vi "2B Dialog with Font Size control.vi"(8 "error in (no error)":errorcluster, 9 "F Button Name (\"Cancel\")":string="Cancel", 10 "T Button Name (\"OK\")":string="Retry", 11 "message":string="System On Signal Not Received.\nPlease TURN ON the System On Switch On the Front Door.") -> (0 "error out":errorcluster, 3 "OK":bool)   [LabVIEW 2018]
panel:
  out "message":string
  in  "OK":bool
  in  "Cancel":bool
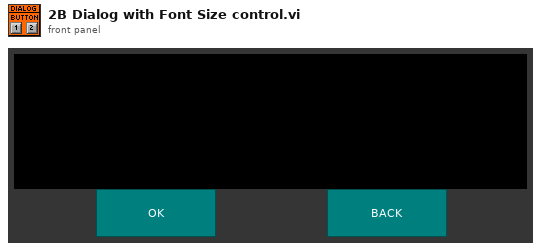
[diagram p1: front panel]
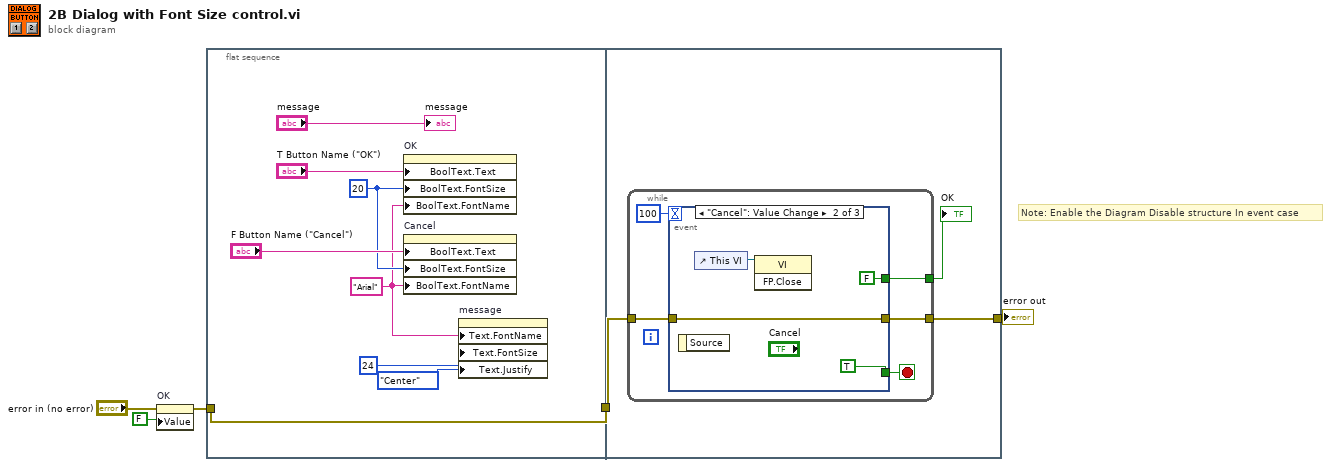
[diagram p0: block diagram]
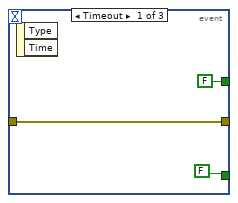
[diagram p2: hidden frame]
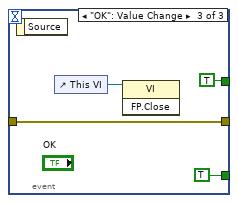
[diagram p3: hidden frame]
diagram:
  # "Note: Enable the Diagram Disable structure In event case"
  n1 = property on="OK" class="Bool (strict)"(error in="error in (no error)", "Value"=FALSE ("OK")) -> (error out=w2:errorcluster)  [unwired: 1 in, 1 out]
  n2 = flat-sequence {
    tunnel: [w10] -> w5
    tunnel: w2 -> [w10]
    tunnel: w5 -> [w15]
    tunnel: [w14] -> w4
    frame #0 {
      w7 = "Arial" ("Font Name")
      w11 = u32 20 ("Boolean Text.Font:Size")
      n3 = property on="OK" class="Bool"("BoolText.Text"="T Button Name (\"OK\")", "BoolText.FontSize"=w11, "BoolText.FontName"=w7) -> ()  [unwired: 2 in, 2 out]
      n4 = property on="Cancel" class="Bool"("BoolText.Text"="F Button Name (\"Cancel\")", "BoolText.FontSize"=w11, "BoolText.FontName"=w7) -> ()  [unwired: 2 in, 2 out]
      n5 = property on="message" class="Str"("Text.FontName"=w7, "Text.FontSize"=u32 24 ("Text.Font:Size"), "Text.Justify"=enum16{"Left", "Center", "Right"}."Center" ("Text.Justification")) -> ()  [unwired: 2 in, 2 out]
      "message" <- "message"
    }
    frame #1 {
      n6 = while {
        tunnel: [w19] -> w16
        tunnel: w15 -> [w17]
        tunnel: [w18] -> w14
        stop <- w20 stop-if-true
        n7 = event shown="[1] \"Cancel\": Value Change" {
          selector: _ -> [_ _ _]
          dyn-events: _ -> [_ _ _]
          timeout: 100 -> [_ _ _]
          tunnel: [FALSE TRUE TRUE] -> w20
          tunnel: [FALSE FALSE TRUE] -> w19
          tunnel: [w22 w26 w30] -> w18
          tunnel: w17 -> [w22 w26 w30]
          event Timeout {
            n8 = event-data() -> ()  [unwired: 3 out]
          }
          event "Cancel": Value Change {
            n9 = event-data() -> ()  [unwired: 2 out]
            n10 = control-ref of="This VI"() -> (w25:refnum<vi>)
            n11 = invoke class="VI" method="FP.Close"(reference=w25) -> ()  [unwired: 2 in, 3 out]
          }
          event "OK": Value Change {
            n12 = event-data() -> ()  [unwired: 2 out]
            n13 = control-ref of="This VI"() -> (w29:refnum<vi>)
            n14 = invoke class="VI" method="FP.Close"(reference=w29) -> ()  [unwired: 2 in, 3 out]
          }
        }
      }
      "OK" <- w16
    }
  }
  "error out" <- w4
